vi "基础 4.vi"() -> ()   [LabVIEW 2014]
panel:
  out "数值":dbl
  out "字符串":string
  out "时间标识":timestamp
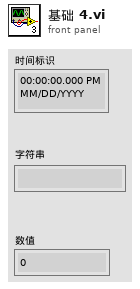
[diagram p1: front panel]
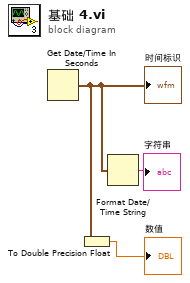
[diagram p0: block diagram]
diagram:
  n1 = Get Date/Time In Seconds() -> (seconds since 1Jan1904=w2:timestamp)
  "时间标识" <- w2
  n2 = To Double Precision Float(number=w2) -> (double precision float=→"数值":dbl)
  n3 = Format Date/Time String(seconds (now)=w2) -> (date/time string=→"字符串":string)  [unwired: 2 in]
